vi "AWG_SequencyRewrite.vi"(8 "error in (no error)":errorcluster, 9 "Value":dbl, 10 "Constant Name":string, 11 "AWG Sequence":string) -> (0 "error out":errorcluster, 3 "result string":string, 5 "number of replacements":i32)   [LabVIEW 2016, in "ZI AWG.lvlib"]
uses:
  <vilib>/Utility/error.llb/whitespace.ctl
  ZI AWG.lvlib
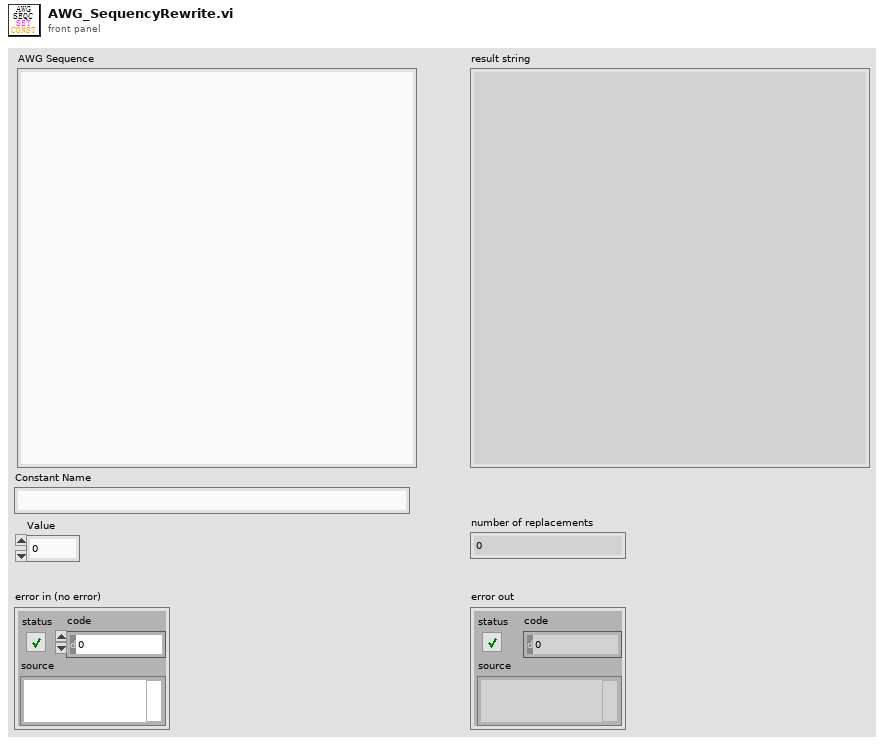
[diagram p1: front panel]
types:
  T1 = typedef "whitespace.ctl" = u16
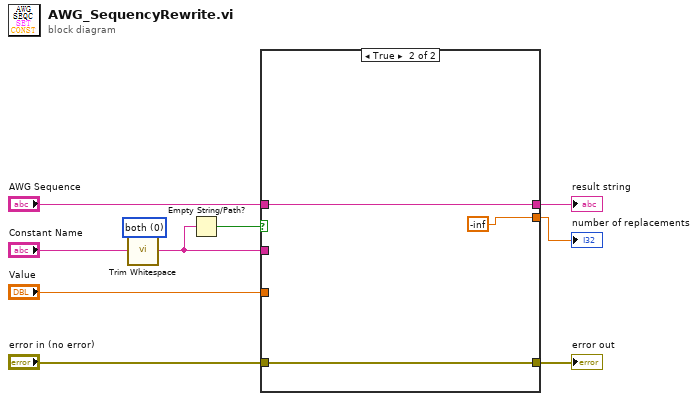
[diagram p0: block diagram]
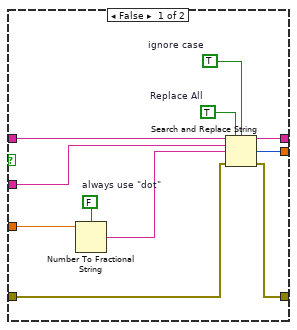
[diagram p2: hidden frame]
diagram:
  w3 = T1 0 items=["both", "start of string", "end of string"] ("location (both)")
  n1 = call <vilib>:"Trim Whitespace.vi"("string"="Constant Name", "location (both)"=w3) -> ("trimmed string"=w2:string)
  n2 = Empty String/Path?(string/path=w2) -> (empty?=w1:bool)
  n3 = case shown="True" w1 {
    tunnel: "AWG Sequence" -> [w21 w24]
    tunnel: [w20 w24] -> w9
    tunnel: "Value" -> [w19 _]
    tunnel: [w14 -inf] -> w7
    tunnel: "error in (no error)" -> [w13 w22]
    tunnel: [w12 w22] -> w5
    tunnel: w2 -> [w11 _]
    frame False {
      w15 = TRUE  # ignore case
      w16 = TRUE  # Replace All
      w18 = FALSE  # always use "dot"
      n4 = Number To Fractional String(use system decimal point (T)=w18, number=w19) -> (F-format string=w17:string)  [unwired: 2 in]
      n5 = Search and Replace String(replace all?=w16, case sensitive?=w15, input string=w21, search string=w11, replace string=w17, error in=w13) -> (result string=w20:string, number of replacements=w14:i32, error out=w12:errorcluster)  [unwired: 2 in, 1 out]
    }
    frame True {
    }
  }
  "result string" <- w9
  "number of replacements" <- w7
  "error out" <- w5
